vi "UTILITY Check Interval.vi"(8 "Error In":errorcluster, 11 "Check Location Interval (Second)":i32) -> (0 "Error Out":errorcluster, 2 "Check Path":bool, 3 "Elapsed Time (sec)":dbl)   [LabVIEW 2016]
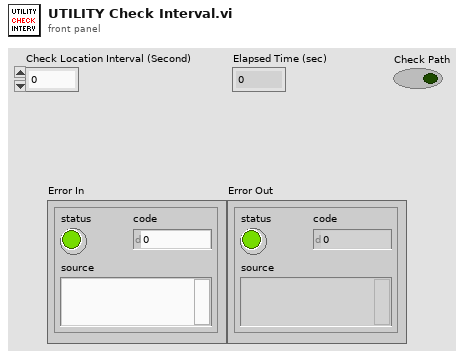
[diagram p1: front panel]
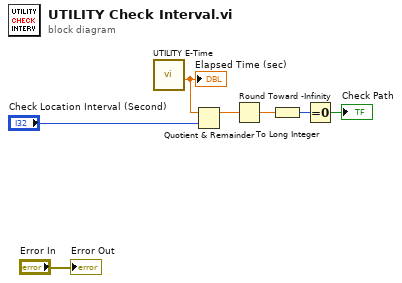
[diagram p0: block diagram]
diagram:
  n1 = call "UTILITY E-Time.vi"() -> ("Elapsed Time (sec)"=w4:dbl)  [unwired: 9 in, 2 out]
  "Elapsed Time (sec)" <- w4
  n2 = Quotient & Remainder(x=w4, y="Check Location Interval (Second)") -> (x-y*floor(x/y)=w2:dbl)  [unwired: 1 out]
  n3 = Round Toward -Infinity(1:w2) -> (0:w1:dbl)
  n4 = To Long Integer(number=w1) -> (32bit integer=w7:i32)
  n5 = Equal To 0?(x=w7) -> (x = 0?=→"Check Path":bool)
  "Error Out" <- "Error In"
